vi "Begin.vi"(8 "error in":errorcluster) -> (0 "error out":errorcluster)   [LabVIEW 2016]
doc: "Called before other user functions, this VI is expected to open initial I/O refnums, load in file data, and do all program initialization. Notice that the <B>error out</B> terminal is simply used for data flow. Wiring it to other structures or subVIs ensures that this VI runs first."
uses:
  <vilib>/Rock Robotics/WPI/DriverStation/WPI_DriverStationRobotMode2.ctl
  <vilib>/Rock Robotics/WPI/ThirdParty/CanMotor/TalonSRX/WPI_CANTalonSRX_APIControlMode.ctl
  <vilib>/Rock Robotics/WPI/ThirdParty/CanMotor/TalonSRX/WPI_CANTalonSRX_APIFeedbackSelect.ctl
  <vilib>/Rock Robotics/WPI/ThirdParty/CanMotor/TalonSRX/WPI_CANTalonSRX_BrakeOverride.ctl
  <vilib>/Rock Robotics/WPI/Joystick/WPI_JoystickDeviceEnum.ctl
  <vilib>/Rock Robotics/WPI/Solenoid/WPI_SolenoidChannel.ctl
  <vilib>/Rock Robotics/SystemInterfaces/DIO/FPGA_DIOPWMChannel.ctl
  <vilib>/Rock Robotics/SystemInterfaces/DIO/FPGA_DIORelayChannel.ctl
  <vilib>/Rock Robotics/WPI/Relay/WPI_RelayDirection.ctl
  Robot Global Data.vi
  <vilib>/Rock Robotics/WPI/Solenoid/WPI_SolenoidOpenDouble.vi
  <vilib>/Rock Robotics/WPI/MotorControl/WPI_MotorControlOpen SPARK.vi
  <vilib>/Rock Robotics/WPI/Utilities/WPI_GetSetVariantRefNum.vi
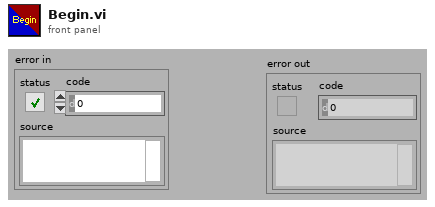
[diagram p1: front panel]
types:
  T1 = typedef "WPI_CANTalonSRX_BrakeOverride.ctl" = enum8{"No Override", "Override to Coast", "Override to Brake"}
  T2 = typedef "WPI_CANTalonSRX_APIControlMode.ctl" = enum8{"Percent VBus", "Speed", "Position", "Slave", "Unchanged / Invalid", "Voltage Compensation", "Current", "Motion Profile", "Motion Magic"}
  T3 = typedef "FPGA_DIOPWMChannel.ctl" = enum8{"PWM 0", "PWM 1", "PWM 2", "PWM 3", "PWM 4", "PWM 5", "PWM 6", "PWM 7", "PWM 8", "PWM 9", "PWM MXP 0", "PWM MXP 1", "PWM MXP 2", "PWM MXP 3", "PWM MXP 4", "PWM MXP 5", "PWM MXP 6", "PWM MXP 7", "PWM MXP 8", "PWM MXP 9", "Invalid"}
  T4 = typedef "WPI_RelayDirection.ctl" = enum16{"Both directions", "Forward only", "Reverse only"}
  T5 = typedef "FPGA_DIORelayChannel.ctl" = enum8{"Relay 0", "Relay 1", "Relay 2", "Relay 3", "Invalid"}
  T6 = typedef "WPI_CANTalonSRX_APIFeedbackSelect.ctl" = enum16{"Digital Quadrature Encoder", "Analog Potentiometer", "Analog Encoder", "Count on Quad-A (Rising-Edge)", "Count on Quad-A (Falling-Edge)", "CTR Magnetic Enc (Absolute)", "CTR Magnetic Enc (Relative)", "Pulse Width"}
  T7 = typedef "WPI_SolenoidChannel.ctl" = enum8{"Solenoid 0", "Solenoid 1", "Solenoid 2", "Solenoid 3", "Solenoid 4", "Solenoid 5", "Solenoid 6", "Solenoid 7", "Invalid"}
  T8 = typedef "WPI_JoystickDeviceEnum.ctl" = enum16{"USB 0", "USB 1", "USB 2", "USB 3", "USB 4", "USB 5"}
  T9 = typedef "WPI_DriverStationRobotMode2.ctl" = enum16{"Autonomous Disabled", "Autonomous Enabled", "Teleop Disabled", "Teleop Enabled", "Disconnected", "Finish", "Test Disabled", "Test Enabled", "Emergency Stopped"}
  T10 = typedef "WPI_MotorControlDeviceRef.ctl" = cluster{"DeviceStatus":errorcluster, "Type":T11, "PWM":cluster{"PWM Channel":T3, "DeadBand":T12}, "CAN":cluster{"Device Number":u8, "SetOutput VI Ref":variant, "GetOutput VI Ref":variant, "Enable VI Ref":variant, "Disable VI Ref":variant, "Data":variant}, "Invert":bool}
  T11 = typedef "WPI_MotorControlType.ctl" = enum16{"PWM", "CAN"}
  T12 = typedef "WPI_PWMDeadband.ctl" = cluster{"Name":string, "maxPositivePwm":i32, "minPositivePwm":i32, "centerPwm":i32, "maxNegativePwm":i32, "minNegativePwm":i32, "angularRange":u16}
  T13 = typedef "WPI_CompressorDevRef.ctl" = cluster{"DevStatus":errorcluster, "Pneumatics Control Module":u8}
  T14 = typedef "WPI_RelayDevRef.ctl" = cluster{"DevStatus":errorcluster, "Relay Channel":T5, "Relay Direction":T4}
  T15 = typedef "WPI_ServoDeviceRef.ctl" = cluster{"DeviceStatus":errorcluster, "PWM Channel":T3, "DeadBand":T12}
  T16 = typedef "WPI_SolenoidDevRef.ctl" = cluster{"DevStatus":errorcluster, "Pneumatics Control Module":u8, "Forward Solenoid Channel":T7, "Reverse Solenoid Channel":T7}
  T17 = typedef "WPI_JoystickDevRef.ctl" = cluster{"Device":T8}
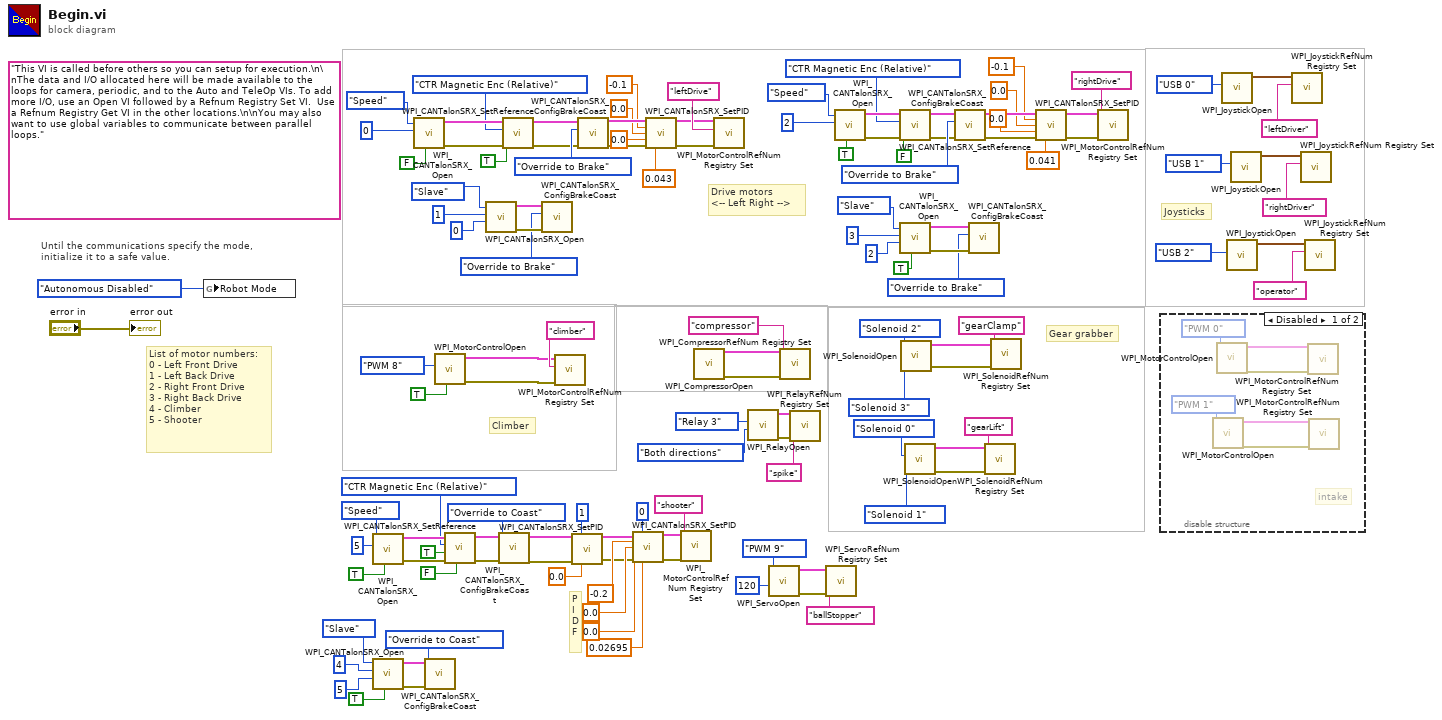
[diagram p0: block diagram]
diagram:
  (unwired) "This VI is called before others so you can setup for execution.\n\nThe data and I/O allocated here will be made available to the loops for camera, periodic, and to the Auto and TeleOp VIs. To add more I/O, use an Open VI followed by a Refnum Registry Set VI.  Use a Refnum Registry Get VI in the other locations.\n\nYou may also want to use global variables to communicate between parallel loops."
  # "P\nI\nD\nF"
  # "List of motor numbers:\n0 - Left Front Drive\n1 - Left Back Drive\n2 - Right Front Drive\n3 - Right Back Drive\n4 - Climber\n5 - Shooter"
  # "Gear grabber"
  # "Joysticks"
  # "Climber"
  # "Drive motors\n<-- Left Right -->"
  # "Until the communications specify the mode,\ninitialize it to a safe value."
  n1 = global write "Robot Global Data.vi" "Robot Mode"(WPI_DriverStationRobotMode2."Autonomous Disabled" ("Robot Mode")) -> ()
  n2 = call <vilib>:"WPI_CANTalonSRX_Open.vi"("Invert"=TRUE, "Device Number"=u8 5, "Control Mode"=WPI_CANTalonSRX_APIControlMode."Speed") -> ("error out"=w42:errorcluster, "CAN Talon SRX Ref"=w43:T10)  [unwired: 7 in]
  n3 = call <vilib>:"WPI_CANTalonSRX_Open.vi"("Invert"=TRUE, "Master Device Number"=u8 5, "Device Number"=u8 4, "Control Mode"=WPI_CANTalonSRX_APIControlMode."Slave") -> ("error out"=w5:errorcluster, "CAN Talon SRX Ref"=w4:T10)  [unwired: 6 in]
  n4 = call <vilib>:"WPI_CANTalonSRX_Open.vi"("Invert"=FALSE, "Device Number"=u8 0, "Control Mode"=WPI_CANTalonSRX_APIControlMode."Speed") -> ("error out"=w117:errorcluster, "CAN Talon SRX Ref"=w118:T10)  [unwired: 7 in]
  n5 = call <vilib>:"WPI_CANTalonSRX_ConfigBrakeCoast.vi"("error in (no error)"=w5, "Brake / Coast Mode"=WPI_CANTalonSRX_BrakeOverride."Override to Coast", "CAN Talon SRX Ref"=w4) -> ()  [unwired: 7 in, 2 out]
  n6 = call-poly <vilib>:"WPI_MotorControlOpen.vi"("Invert"=TRUE, "PWM Channel"=FPGA_DIOPWMChannel."PWM 8") -> ("error out"=w74:errorcluster, "MotorControlDeviceRef"=w75:T10)  [unwired: 8 in]
  n7 = call <vilib>:"WPI_CANTalonSRX_SetReference.vi"("Reverse Closed-Loop Output"=FALSE, "error in (no error)"=w42, "Reverse Feedback Sensor"=TRUE, "Feedback Reference"=WPI_CANTalonSRX_APIFeedbackSelect."CTR Magnetic Enc (Relative)", "CAN Talon SRX Ref"=w43) -> ("error out"=w39:errorcluster, "CAN Talon SRX Ref"=w38:T10)  [unwired: 5 in]
  n8 = call <vilib>:"WPI_CANTalonSRX_Open.vi"("Master Device Number"=u8 0, "Device Number"=u8 1, "Control Mode"=WPI_CANTalonSRX_APIControlMode."Slave") -> ("error out"=w109:errorcluster, "CAN Talon SRX Ref"=w110:T10)  [unwired: 7 in]
  n9 = call <vilib>:"WPI_CANTalonSRX_ConfigBrakeCoast.vi"("error in (no error)"=w39, "Brake / Coast Mode"=WPI_CANTalonSRX_BrakeOverride."Override to Coast", "CAN Talon SRX Ref"=w38) -> ("error out"=w17:errorcluster, "CAN Talon SRX Ref"=w20:T10)  [unwired: 7 in]
  n10 = call <vilib>:"WPI_CANTalonSRX_SetReference.vi"("error in (no error)"=w117, "Reverse Feedback Sensor"=TRUE, "Feedback Reference"=WPI_CANTalonSRX_APIFeedbackSelect."CTR Magnetic Enc (Relative)", "CAN Talon SRX Ref"=w118) -> ("error out"=w114:errorcluster, "CAN Talon SRX Ref"=w113:T10)  [unwired: 6 in]
  n11 = call <vilib>:"WPI_CANTalonSRX_ConfigBrakeCoast.vi"("error in (no error)"=w109, "Brake / Coast Mode"=WPI_CANTalonSRX_BrakeOverride."Override to Brake", "CAN Talon SRX Ref"=w110) -> ()  [unwired: 7 in, 2 out]
  n12 = call <vilib>:"WPI_MotorControlRefNum Registry Set.vi"("error in (no error)"=w74, "refnum name"="climber", "MotorControlDevRef"=w75) -> ()  [unwired: 7 in, 2 out]
  n13 = call <vilib>:"WPI_CANTalonSRX_SetPID.vi"("CAN Talon SRX Ref"=w20, "Parameter Slot"=u8 1, "error in (no error)"=w17, "F"=0.0) -> ("CAN Talon SRX Ref"=w19:T10, "error out"=w18:errorcluster)  [unwired: 10 in]
  n14 = call <vilib>:"WPI_CANTalonSRX_ConfigBrakeCoast.vi"("error in (no error)"=w114, "Brake / Coast Mode"=WPI_CANTalonSRX_BrakeOverride."Override to Brake", "CAN Talon SRX Ref"=w113) -> ("error out"=w73:errorcluster, "CAN Talon SRX Ref"=w71:T10)  [unwired: 7 in]
  n15 = call <vilib>:"WPI_CANTalonSRX_SetPID.vi"("CAN Talon SRX Ref"=w19, "Parameter Slot"=u8 0, "P"=-0.2, "I"=0.0, "D"=0.0, "error in (no error)"=w18, "F"=0.02695) -> ("CAN Talon SRX Ref"=w24:T10, "error out"=w23:errorcluster)  [unwired: 7 in]
  n16 = call <vilib>:"WPI_CANTalonSRX_SetPID.vi"("CAN Talon SRX Ref"=w71, "P"=-0.1, "I"=0.0, "D"=0.0, "error in (no error)"=w73, "F"=0.043) -> ("CAN Talon SRX Ref"=w70:T10, "error out"=w72:errorcluster)  [unwired: 8 in]
  n17 = call <vilib>:"WPI_MotorControlRefNum Registry Set.vi"("error in (no error)"=w23, "refnum name"="shooter", "MotorControlDevRef"=w24) -> ()  [unwired: 7 in, 2 out]
  n18 = call <vilib>:"WPI_CompressorOpen.vi"() -> ("CompressorDevRef"=w57:T13, "error out"=w56:errorcluster)  [unwired: 14 in]
  n19 = call <vilib>:"WPI_MotorControlRefNum Registry Set.vi"("error in (no error)"=w72, "refnum name"="leftDrive", "MotorControlDevRef"=w70) -> ()  [unwired: 7 in, 2 out]
  n20 = call <vilib>:"WPI_RelayOpen.vi"("Relay Direction"=WPI_RelayDirection."Both directions", "Relay Channel"=FPGA_DIORelayChannel."Relay 3") -> ("error out"=w13:errorcluster, "RelayDevRef"=w14:T14)  [unwired: 8 in]
  n21 = call <vilib>:"WPI_ServoOpen.vi"("Angular Range"=u16 120, "PWM Channel"=FPGA_DIOPWMChannel."PWM 9") -> ("error out"=w30:errorcluster, "ServoDeviceRef"=w29:T15)  [unwired: 8 in]
  n22 = call <vilib>:"WPI_CompressorRefNum Registry Set.vi"("error in (no error)"=w56, "refnum name"="compressor", "CompressorDevRef"=w57) -> ()  [unwired: 7 in, 2 out]
  n23 = call <vilib>:"WPI_RelayRefNum Registry Set.vi"("error in (no error)"=w13, "refnum name"="spike", "RelayDevRef"=w14) -> ()  [unwired: 7 in, 2 out]
  n24 = call <vilib>:"WPI_ServoRefNum Registry Set.vi"("error in (no error)"=w30, "refnum name"="ballStopper", "ServoDeviceRef"=w29) -> ()  [unwired: 7 in, 2 out]
  n25 = call <vilib>:"WPI_CANTalonSRX_Open.vi"("Invert"=TRUE, "Device Number"=u8 2, "Control Mode"=WPI_CANTalonSRX_APIControlMode."Speed") -> ("error out"=w103:errorcluster, "CAN Talon SRX Ref"=w104:T10)  [unwired: 7 in]
  n26 = call <vilib>:"WPI_CANTalonSRX_SetReference.vi"("error in (no error)"=w103, "Reverse Feedback Sensor"=FALSE, "Feedback Reference"=WPI_CANTalonSRX_APIFeedbackSelect."CTR Magnetic Enc (Relative)", "CAN Talon SRX Ref"=w104) -> ("error out"=w100:errorcluster, "CAN Talon SRX Ref"=w99:T10)  [unwired: 6 in]
  n27 = call <vilib>:"WPI_CANTalonSRX_Open.vi"("Invert"=TRUE, "Master Device Number"=u8 2, "Device Number"=u8 3, "Control Mode"=WPI_CANTalonSRX_APIControlMode."Slave") -> ("error out"=w94:errorcluster, "CAN Talon SRX Ref"=w95:T10)  [unwired: 6 in]
  n28 = call-poly <vilib>:"WPI_SolenoidOpen.vi"("Reverse Solenoid Channel"=WPI_SolenoidChannel."Solenoid 3", "Forward Solenoid Channel"=WPI_SolenoidChannel."Solenoid 2") -> ("error out"=w47:errorcluster, "SolenoidDevRef"=w48:T16)  [unwired: 8 in]
  n29 = call-poly <vilib>:"WPI_SolenoidOpen.vi"("Reverse Solenoid Channel"=WPI_SolenoidChannel."Solenoid 1", "Forward Solenoid Channel"=WPI_SolenoidChannel."Solenoid 0") -> ("error out"=w49:errorcluster, "SolenoidDevRef"=w50:T16)  [unwired: 8 in]
  n30 = call <vilib>:"WPI_CANTalonSRX_ConfigBrakeCoast.vi"("error in (no error)"=w100, "Brake / Coast Mode"=WPI_CANTalonSRX_BrakeOverride."Override to Brake", "CAN Talon SRX Ref"=w99) -> ("error out"=w62:errorcluster, "CAN Talon SRX Ref"=w65:T10)  [unwired: 7 in]
  n31 = call <vilib>:"WPI_CANTalonSRX_ConfigBrakeCoast.vi"("error in (no error)"=w94, "Brake / Coast Mode"=WPI_CANTalonSRX_BrakeOverride."Override to Brake", "CAN Talon SRX Ref"=w95) -> ()  [unwired: 7 in, 2 out]
  n32 = call <vilib>:"WPI_SolenoidRefNum Registry Set.vi"("error in (no error)"=w49, "refnum name"="gearLift", "SolenoidDevRef"=w50) -> ()  [unwired: 7 in, 2 out]
  n33 = call <vilib>:"WPI_SolenoidRefNum Registry Set.vi"("error in (no error)"=w47, "refnum name"="gearClamp", "SolenoidDevRef"=w48) -> ()  [unwired: 7 in, 2 out]
  n34 = call <vilib>:"WPI_CANTalonSRX_SetPID.vi"("CAN Talon SRX Ref"=w65, "P"=-0.1, "I"=0.0, "D"=0.0, "error in (no error)"=w62, "F"=0.041) -> ("CAN Talon SRX Ref"=w64:T10, "error out"=w63:errorcluster)  [unwired: 8 in]
  n35 = call <vilib>:"WPI_MotorControlRefNum Registry Set.vi"("error in (no error)"=w63, "refnum name"="rightDrive", "MotorControlDevRef"=w64) -> ()  [unwired: 7 in, 2 out]
  n36 = disable-structure shown="Disabled" {
    frame Disabled {
      # "intake"
      n37 = call-poly <vilib>:"WPI_MotorControlOpen.vi"("PWM Channel"=FPGA_DIOPWMChannel."PWM 1") -> ("error out"=w123:errorcluster, "MotorControlDeviceRef"=w124:T10)  [unwired: 9 in]
      n38 = call-poly <vilib>:"WPI_MotorControlOpen.vi"("PWM Channel"=FPGA_DIOPWMChannel."PWM 0") -> ("error out"=w125:errorcluster, "MotorControlDeviceRef"=w126:T10)  [unwired: 9 in]
      n39 = call <vilib>:"WPI_MotorControlRefNum Registry Set.vi"("error in (no error)"=w125, "MotorControlDevRef"=w126) -> ()  [unwired: 8 in, 2 out]
      n40 = call <vilib>:"WPI_MotorControlRefNum Registry Set.vi"("error in (no error)"=w123, "MotorControlDevRef"=w124) -> ()  [unwired: 8 in, 2 out]
    }
    frame Enabled {
    }
  }
  n41 = call <vilib>:"WPI_JoystickOpen.vi"("JoystickDevice"=WPI_JoystickDeviceEnum."USB 0") -> ("JoystickDevRef"=w90:T17)  [unwired: 10 in]
  n42 = call <vilib>:"WPI_JoystickOpen.vi"("JoystickDevice"=WPI_JoystickDeviceEnum."USB 2") -> ("JoystickDevRef"=w79:T17)  [unwired: 10 in]
  n43 = call <vilib>:"WPI_JoystickOpen.vi"("JoystickDevice"=WPI_JoystickDeviceEnum."USB 1") -> ("JoystickDevRef"=w87:T17)  [unwired: 10 in]
  n44 = call <vilib>:"WPI_JoystickRefNum Registry Set.vi"("refnum name"="leftDriver", "JoystickDevRef"=w90) -> ()  [unwired: 8 in, 2 out]
  n45 = call <vilib>:"WPI_JoystickRefNum Registry Set.vi"("refnum name"="rightDriver", "JoystickDevRef"=w87) -> ()  [unwired: 8 in, 2 out]
  n46 = call <vilib>:"WPI_JoystickRefNum Registry Set.vi"("refnum name"="operator", "JoystickDevRef"=w79) -> ()  [unwired: 8 in, 2 out]
  "error out" <- "error in"
